vi "PM100-Get Range.vi"(0 "VISA in":refnum<visa-resource-name>, 7 "Power (W)":dbl, 11 "error in (no error)":errorcluster) -> (4 "VISA out":refnum<visa-resource-name>, 8 "lblRange":string, 15 "error out":errorcluster)   [LabVIEW 2015]
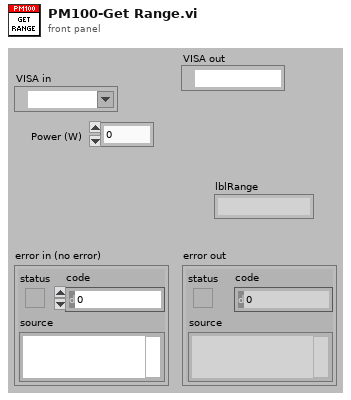
[diagram p1: front panel]
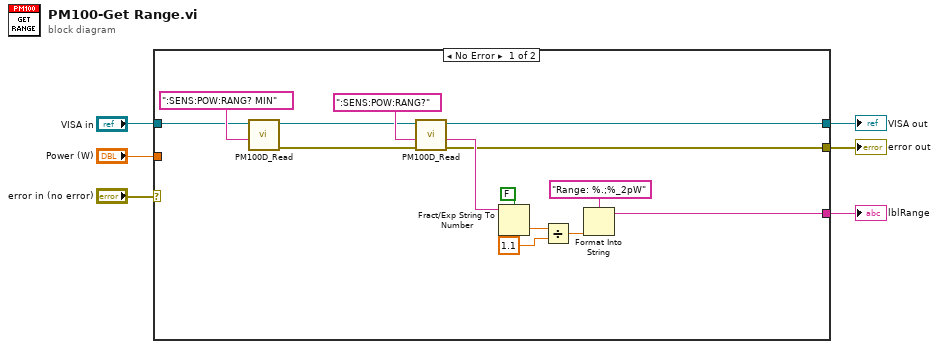
[diagram p0: block diagram]
diagram:
  n1 = case shown="No Error" "error in (no error)" {
    selector: "error in (no error)" -> [_ w22]
    tunnel: "VISA in" -> [w9 w21]
    tunnel: [w12 w22] -> w4
    tunnel: "Power (W)" -> [_ _]
    tunnel: [w14 w21] -> w2
    tunnel: [w11 _] -> w1
    frame No Error {
      n2 = call "PM100D_Read.vi"("Command"=":SENS:POW:RANG? MIN", "VISA in"=w9) -> ("error out"=w7:errorcluster, "VISA out"=w8:refnum<visa-resource-name>)  [unwired: 7 in, 1 out]
      n3 = call "PM100D_Read.vi"("error in (no error)"=w7, "Command"=":SENS:POW:RANG?", "VISA in"=w8) -> ("error out"=w12:errorcluster, "ReadValue"=w13:string, "VISA out"=w14:refnum<visa-resource-name>)  [unwired: 6 in]
      n4 = Fract/Exp String To Number(use system decimal point (T)=FALSE, string=w13) -> (number=w16:dbl)  [unwired: 2 in, 1 out]
      n5 = Divide(x=w16, y=1.1) -> (x/y=w18:dbl)
      n6 = Format Into String(format string="Range: %.;%_2pW", w18) -> (resulting string=w11:string)  [unwired: 2 in, 1 out]
    }
    frame Error {
    }
  }
  "error out" <- w4
  "VISA out" <- w2
  "lblRange" <- w1
